vi "target - single rate - variables.vi"() -> ()   [LabVIEW 2017]
uses:
  <vilib>/Platform/TimedLoop/XDataNode/timing_clust.ctl
  <vilib>/Platform/TimedLoop/XDataNode/nitl_modes.ctl
  <vilib>/Platform/TimedLoop/XDataNode/wakeup.ctl
  <vilib>/Platform/TimedLoop/XDataNode/XDataNode.xnode
  <vilib>/Platform/TimedLoop/XDataNode/XDNodeRunTimeDep.lvlib
panel:
  out "error out":errorcluster
  out "error Mesurment":errorcluster
  out "error IO":errorcluster
  out "value":dbl
  in  "stop":bool
  out "Loop counter":i32
  in  "On/~Off":bool
  in  "Enable/~Disable":bool
  in  "Forward/~Backward":bool
  out "State":bool[](array[boolean])
  # "The Network Variable Engine and Variable Client Support must be installed on the RT target\nfor this application to function properly. If the Network Variable Engine is not supported on\nthe target (e.g.  FP-2000 with <32MB of RAM), open the project and move the variable library\nto My Computer in the project. Doing this will deploy the variables to localhost but\nwill still require that Variable Client Support be installed on the RT target."
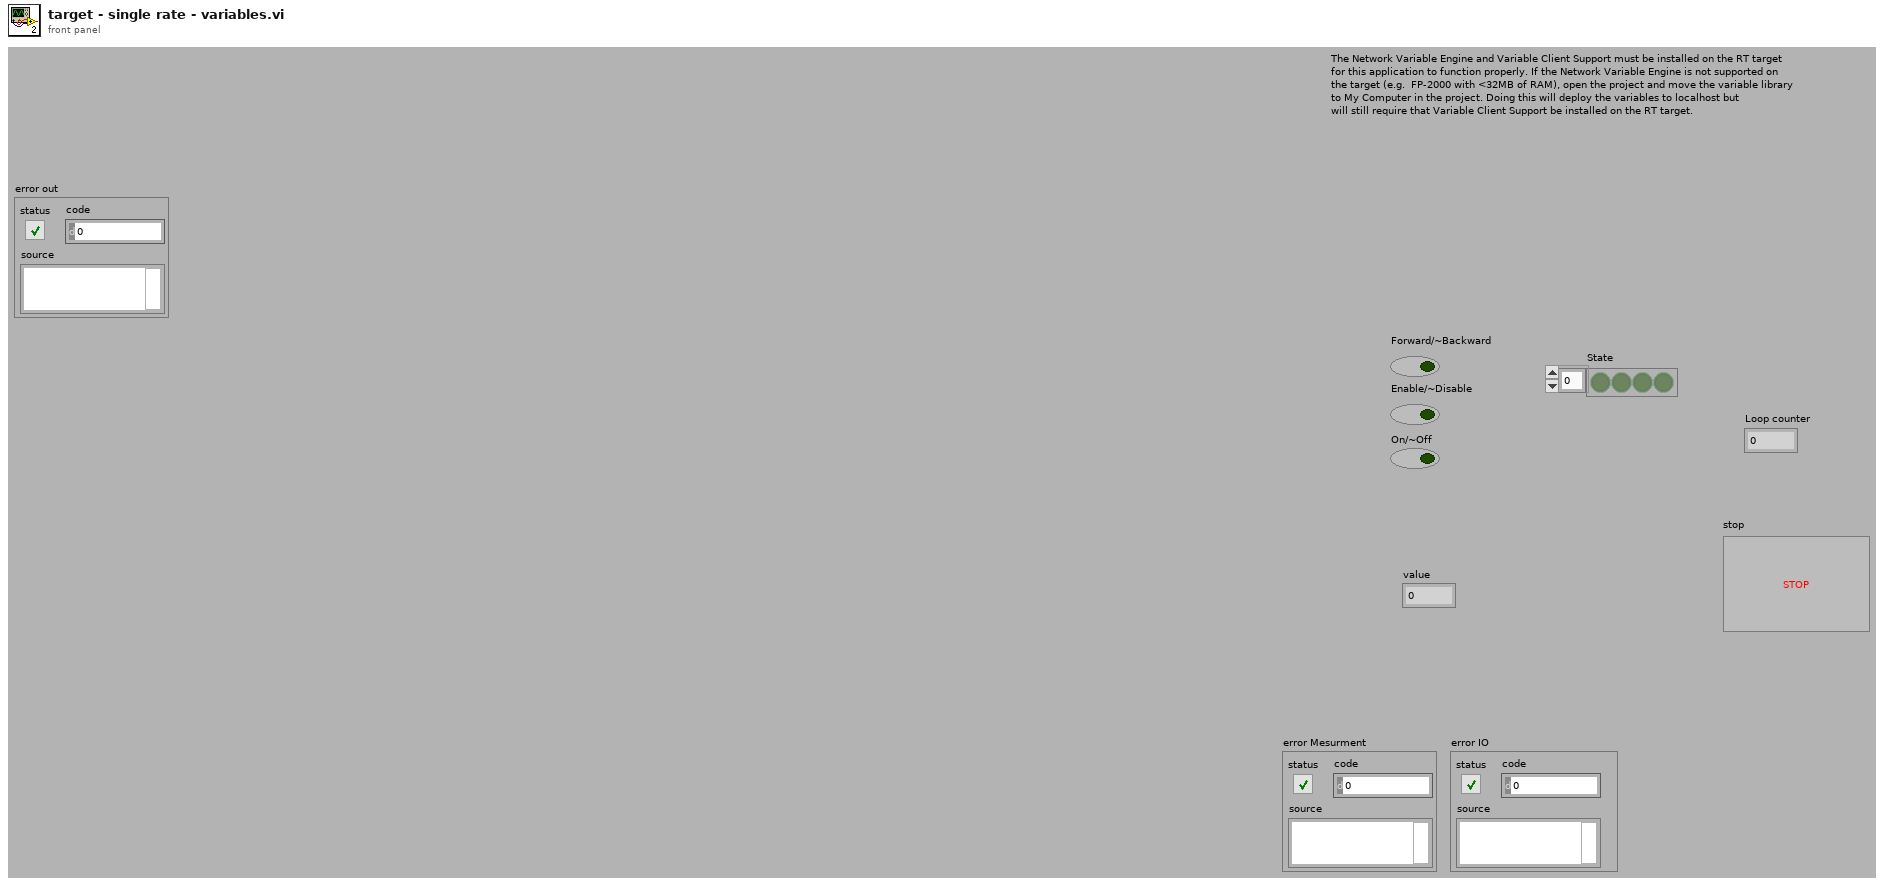
[diagram p1: front panel]
types:
  T1 = typedef "XDNodeRunTimeDep.lvlib/timing_clust.ctl" = cluster{"Expected End [f-1]":u64, "Actual End [f-1]":u64, "Finished Late? [f-1]":bool, "Expected End [i-1]":u64, "Actual End [i-1]":u64, "Finished Late? [i-1]":bool, "Expected Start [i]":u64, "Actual Start [i]":u64, "Expected Start [f]":u64, "Actual Start [f]":u64, "Source Name":string, "Structure Name":string, "Period":i64, "Deadline":i64, "Offset":i64, "Start":i64, "Priority":i32, "Timeout":i32, "Mode":T2, "Wakeup Reason":T3, "Error":errorcluster, "Source Type":string, "Secondary Source Type":string, "Global End Time":u64, "Global Start Time":u64, "Frame Duration":u64, "Iteration Duration":u64, "Assigned CPU":i32, "I/O Scan Engine Mode":u32}
  T2 = typedef "XDNodeRunTimeDep.lvlib/nitl_modes.ctl" = enum32{"No Change", "Process missed periods, maintain original phase", "Discard missed periods, maintain original phase", "Process missed periods, ignore original phase", "Discard missed periods, ignore original phase"}
  T3 = typedef "XDNodeRunTimeDep.lvlib/wakeup.ctl" = enum32{"Normal", "Aborted", "Asynchronous wakeup", "Timing source error", "Timed loop error", "Timeout"}
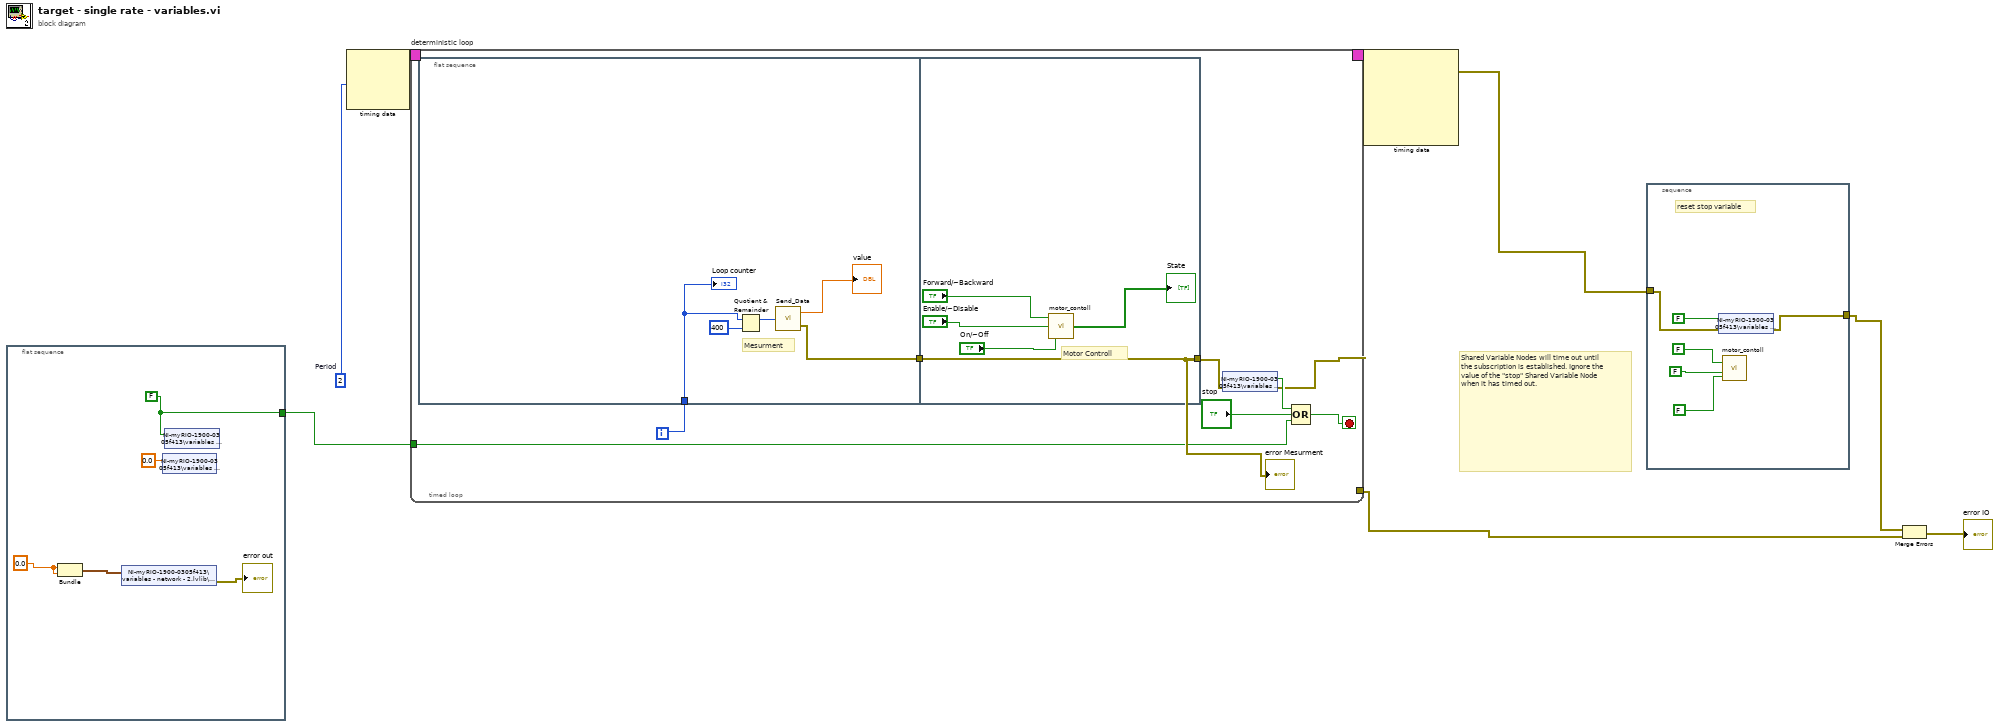
[diagram p0: block diagram]
diagram:
  w6 = i64 2  # Period
  # "Shared Variable Nodes will time out until the subscription is established. Ignore the value of the \"stop\" Shared Variable Node when it has timed out."
  n1 = flat-sequence {
    tunnel: [w13] -> w1
    frame #0 {
      w9 = 0.0 ("data")
      w13 = FALSE ("stop")
      n2 = Bundle("data"=w9, "data"=w9) -> (w10:cluster{"data":dbl, "data":dbl})  [unwired: 1 in]
      n3 = shared-variable "NI-myRIO-1900-0305f413\\variables - network - 2.lvlib\\output cluster"(w10) -> (error out=→"error out":errorcluster)  [unwired: 1 in]
      n4 = shared-variable "NI-myRIO-1900-0305f413\\variables - network - RT.lvlib\\data"(0.0 ("data")) -> ()  [unwired: 1 in, 1 out]
      n5 = shared-variable "NI-myRIO-1900-0305f413\\variables - network - RT.lvlib\\stop"(w13) -> ()  [unwired: 1 in, 1 out]
    }
  }
  n6 = node-c288 ("Input Node")(w6) -> (w8:T1)  [unwired: 2 in]
  n7 = timed-loop "deterministic loop" {
    timing: w8 -> [_]
    timing-out: [_] -> w7
    tunnel: [w16] -> w2
    tunnel: w1 -> [w14]
    i -> [w18]
    stop <- w21 stop-if-true
    # "Motor Controll"
    n8 = flat-sequence {
      tunnel: w18 -> [w24]
      tunnel: [w23] -> w17
      tunnel: [w31] -> w15
      tunnel: w17 -> [w31]
      frame #0 {
        # "Mesurment"
        n9 = Quotient & Remainder(x=w24, y=400) -> (x-y*floor(x/y)=w22:i32)  [unwired: 1 out]
        n10 = call "Send_Data.vi"("Poss"=w22) -> ("value"=→"value":dbl, "error out"=w23:errorcluster)
        "Loop counter" <- w24
      }
      frame #1 {
        n11 = call "motor_contoll.vi"("On/Off"="On/~Off", "Enable/Disable"="Enable/~Disable", "Forward/Backward"="Forward/~Backward") -> ("State"=→"State":bool[])
      }
    }
    n12 = shared-variable "NI-myRIO-1900-0305f413\\variables - network - RT.lvlib\\stop"(error in=w15) -> (w19:bool, error out=w16:errorcluster)
    n13 = Compound Arithmetic op=OR(w19, "stop", w14) -> (w21:bool)
    "error Mesurment" <- w15
  }
  n14 = node-c288 ("Output Node")(w7) -> (w5:errorcluster)  [unwired: 5 out]
  n15 = stacked-sequence {
    tunnel: w5 -> [w34]
    tunnel: [w35] -> w3
    frame #0 {
      # "reset stop variable"
      n16 = shared-variable "NI-myRIO-1900-0305f413\\variables - network - RT.lvlib\\stop"(FALSE, error in=w34) -> (error out=w35:errorcluster)
      n17 = call "motor_contoll.vi"("On/Off"=FALSE ("On/~Off"), "Enable/Disable"=FALSE ("Enable/~Disable"), "Forward/Backward"=FALSE ("Forward/~Backward")) -> ()  [unwired: 1 out]
    }
  }
  n18 = Merge Errors(w3, w2) -> (→"error IO":errorcluster)
